vi "SocketHandle_1 - 複製.vi"(7 "Mode":enum16{"Open", "Read", "Write", "Close"}(ring), 8 "error in (no error)":errorcluster, 9 "data in":string, 10 "Port":u16=6342, 11 "Machine":string="localhost") -> (0 "error out":errorcluster, 3 "data out":string)   [LabVIEW 2011]
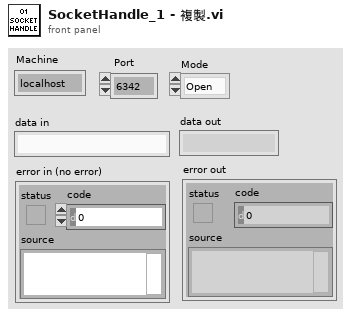
[diagram p1: front panel]
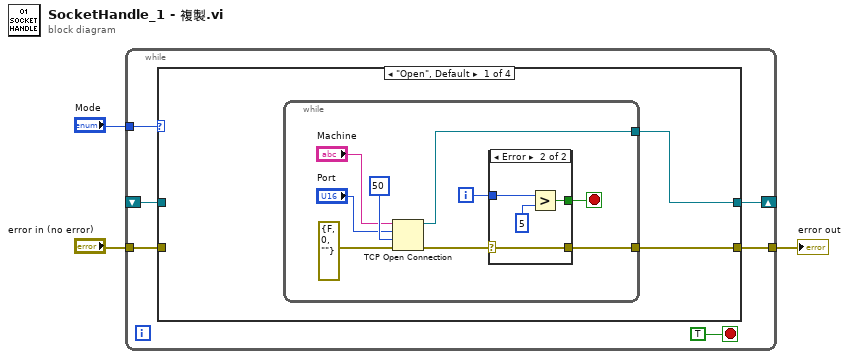
[diagram p0: block diagram]
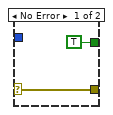
[diagram p2: hidden frame]
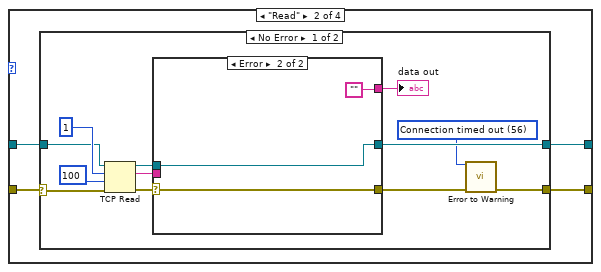
[diagram p3: hidden frame]
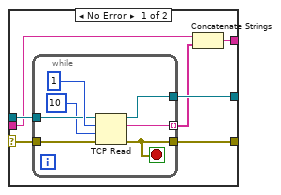
[diagram p4: hidden frame]
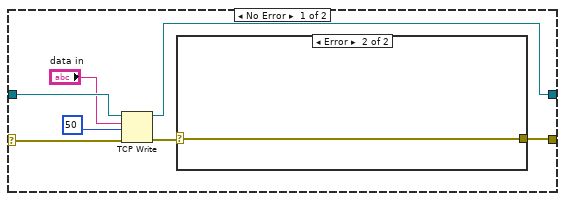
[diagram p7: hidden frame]
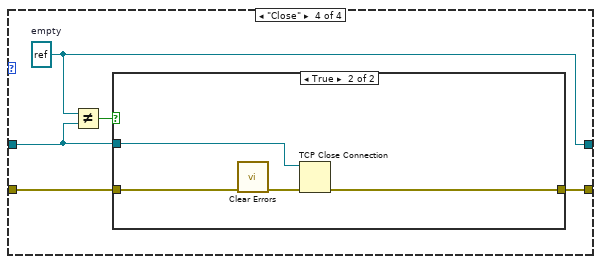
[diagram p9: hidden frame]
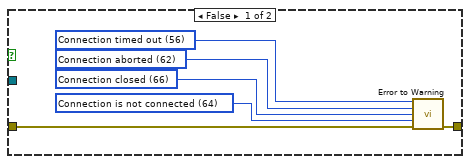
[diagram p10: hidden frame]
diagram:
  n1 = while {
    shift-right: [w9] -> _
    shift-left: _ -> [w6]
    tunnel: "Mode" -> [w5]
    tunnel: "error in (no error)" -> [w7]
    tunnel: [w8] -> w1
    stop <- TRUE stop-if-true
    n2 = case shown="\"Open\", Default" w5 {
      tunnel: [w11 w30 w64 w77] -> w9
      tunnel: [w10 w27 w63 w81] -> w8
      tunnel: w7 -> [_ w28 w62 w80]
      tunnel: w6 -> [_ w29 w65 w78]
      frame "Open", Default {
        n3 = while {
          tunnel: [w20] -> w11
          tunnel: [w15] -> w10
          i -> [w13]
          stop <- w12 stop-if-true
          n4 = TCP Open Connection(address="Machine", remote port or service name="Port", timeout ms (60000)=50, error in (no error)=errorcluster {"status"=FALSE, "code"=0, "source"=""} ("error constant")) -> (connection ID=w20:refnum<k5>, error out=w14:errorcluster)  [unwired: 1 out]
          n5 = case shown="Error" w14 {
            selector: w14 -> [w21 w26]
            tunnel: [w21 w26] -> w15
            tunnel: w13 -> [_ w25]
            tunnel: [TRUE w23] -> w12
            frame No Error {
            }
            frame Error {
              n6 = Greater?(x=w25, y=5) -> (0:w23:bool)
            }
          }
        }
      }
      frame "Read" {
        n7 = case shown="No Error" w28 {
          selector: w28 -> [w34 w60]
          tunnel: [w31 w60] -> w27
          tunnel: [w37 w61] -> w30
          tunnel: w29 -> [w36 w61]
          frame No Error {
            w33 = 56 items=["No Error", "Argument Error", "Memory Full", "Out of Zone", "End of File", "File Already Open", "Generic File IO Error", "File Not Found", "File Permission Error", "Disk Full", "Duplicate Path", "Too Many Files Open", "Not Enabled", "Resource File Not Found", "Cannot Add Resource", "Resource Not Found", "Image Not Found", "Image Memory Error", "Pen Does Not Exist", "Config Bad Type", "Config Token Not Found", "Config Parse Error", "Config Memory Error", "Bad External Code Format", "Bad External Code Offset", "External Code Not Present", "Null Window", "Destroy Window Mixup", "Null Menu", "Print Aborted", "Bad Print Record", "Print Driver Error", "Windows Error During Print", "Memory Error During Print", "Print Dialog Error", "Generic Print Error", "Invalid Device Refnum", "Device Not Found", "Device Parameter Error", "Device Unit Error", "Can't Open Device", "Device Call Aborted", "Generic Error", "Cancelled By User", "Object ID Too Low", "Object ID Too High", "Object Not In Heap", "Unknown Heap", "Bad DefProc ID", "DefProc Not In Table", "Message Out Of Range", "Null Method", "Unknown Message", "Manager Call Not Supported", "Bad address", "Connection In progress", "Connection timed out", "Connection is already in progress", "Network attribute not supported", "Network error", "Address in use", "System out of memory", "Connection aborted", "Connection refused", "Connection is not connected", "Connection is already connected", "Connection closed", "Initialize error (interapplication manager)", "Bad occurrence", "Wait on unbound occurrence handler", "Occurrence queue overflow", "Bad path", "Semaphore not signaled", "Unrecognized type (interapplication manager)"] ("1st Error to Convert")
            n8 = TCP Read(connection ID=w36, bytes to read=1, error in (no error)=w34, 9:100 ("timeout ms (25000)")) -> (connection ID out=w41:refnum<k5>, data out=w42:string, error out=w39:errorcluster)  [unwired: 1 in]
            n9 = case shown="Error" w39 {
              selector: w39 -> [w49 w58]
              tunnel: w42 -> [w44 _]
              tunnel: w41 -> [w48 w59]
              tunnel: [w47 w59] -> w37
              tunnel: [w46 ""] -> w35
              tunnel: [w43 w58] -> w32
              frame No Error {
                n10 = while {
                  tunnel: w49 -> [w56]
                  tunnel: w48 -> [w54]
                  tunnel: [w53] -> w47
                  tunnel: [w52] -> w45 mode=indexing
                  tunnel: [w51] -> w43
                  stop <- w51 stop-if-true
                  n11 = TCP Read(connection ID=w54, bytes to read=1, error in (no error)=w56, 9:10 ("timeout ms (25000)")) -> (connection ID out=w53:refnum<k5>, data out=w52:string, error out=w51:errorcluster)  [unwired: 1 in]
                }
                n12 = Concatenate Strings(w44, w45) -> (w46:string)
              }
              frame Error {
              }
            }
            "data out" <- w35
            n13 = call <vilib>:"Error to Warning.vi"("1st Error to Convert"=w33, "error in"=w32) -> ("warning out"=w31:errorcluster)  [unwired: 13 in]
          }
          frame Error {
          }
        }
      }
      frame "Write" {
        n14 = case shown="Error" w62 {
          selector: w62 -> [w70 w75]
          tunnel: w65 -> [w72 w76]
          tunnel: [w66 w76] -> w64
          tunnel: [w67 w75] -> w63
          frame No Error {
            n15 = TCP Write(connection ID=w72, data in="data in", error in (no error)=w70, 9:50 ("timeout ms (25000)")) -> (connection ID out=w66:refnum<k5>, error out=w68:errorcluster)  [unwired: 1 out]
            n16 = case shown="Error" w68 {
              selector: w68 -> [w73 w74]
              tunnel: [w73 w74] -> w67
              frame No Error {
              }
              frame Error {
              }
            }
          }
          frame Error {
          }
        }
      }
      frame "Close" {
        w77 = refnum<k5> refnum  # empty
        n17 = Not Equal?(x=w77, y=w78) -> (x != y?=w79:bool)
        n18 = case shown="True" w79 {
          tunnel: [w86 w91] -> w81
          tunnel: w80 -> [w87 w90]
          tunnel: w78 -> [_ w88]
          frame False {
            w82 = 64 items=["No Error", "Argument Error", "Memory Full", "Out of Zone", "End of File", "File Already Open", "Generic File IO Error", "File Not Found", "File Permission Error", "Disk Full", "Duplicate Path", "Too Many Files Open", "Not Enabled", "Resource File Not Found", "Cannot Add Resource", "Resource Not Found", "Image Not Found", "Image Memory Error", "Pen Does Not Exist", "Config Bad Type", "Config Token Not Found", "Config Parse Error", "Config Memory Error", "Bad External Code Format", "Bad External Code Offset", "External Code Not Present", "Null Window", "Destroy Window Mixup", "Null Menu", "Print Aborted", "Bad Print Record", "Print Driver Error", "Windows Error During Print", "Memory Error During Print", "Print Dialog Error", "Generic Print Error", "Invalid Device Refnum", "Device Not Found", "Device Parameter Error", "Device Unit Error", "Can't Open Device", "Device Call Aborted", "Generic Error", "Cancelled By User", "Object ID Too Low", "Object ID Too High", "Object Not In Heap", "Unknown Heap", "Bad DefProc ID", "DefProc Not In Table", "Message Out Of Range", "Null Method", "Unknown Message", "Manager Call Not Supported", "Bad address", "Connection In progress", "Connection timed out", "Connection is already in progress", "Network attribute not supported", "Network error", "Address in use", "System out of memory", "Connection aborted", "Connection refused", "Connection is not connected", "Connection is already connected", "Connection closed", "Initialize error (interapplication manager)", "Bad occurrence", "Wait on unbound occurrence handler", "Occurrence queue overflow", "Bad path", "Semaphore not signaled", "Unrecognized type (interapplication manager)"] ("1st Error to Convert")
            w83 = 66 items=["No Error", "Argument Error", "Memory Full", "Out of Zone", "End of File", "File Already Open", "Generic File IO Error", "File Not Found", "File Permission Error", "Disk Full", "Duplicate Path", "Too Many Files Open", "Not Enabled", "Resource File Not Found", "Cannot Add Resource", "Resource Not Found", "Image Not Found", "Image Memory Error", "Pen Does Not Exist", "Config Bad Type", "Config Token Not Found", "Config Parse Error", "Config Memory Error", "Bad External Code Format", "Bad External Code Offset", "External Code Not Present", "Null Window", "Destroy Window Mixup", "Null Menu", "Print Aborted", "Bad Print Record", "Print Driver Error", "Windows Error During Print", "Memory Error During Print", "Print Dialog Error", "Generic Print Error", "Invalid Device Refnum", "Device Not Found", "Device Parameter Error", "Device Unit Error", "Can't Open Device", "Device Call Aborted", "Generic Error", "Cancelled By User", "Object ID Too Low", "Object ID Too High", "Object Not In Heap", "Unknown Heap", "Bad DefProc ID", "DefProc Not In Table", "Message Out Of Range", "Null Method", "Unknown Message", "Manager Call Not Supported", "Bad address", "Connection In progress", "Connection timed out", "Connection is already in progress", "Network attribute not supported", "Network error", "Address in use", "System out of memory", "Connection aborted", "Connection refused", "Connection is not connected", "Connection is already connected", "Connection closed", "Initialize error (interapplication manager)", "Bad occurrence", "Wait on unbound occurrence handler", "Occurrence queue overflow", "Bad path", "Semaphore not signaled", "Unrecognized type (interapplication manager)"] ("1st Error to Convert")
            w84 = 62 items=["No Error", "Argument Error", "Memory Full", "Out of Zone", "End of File", "File Already Open", "Generic File IO Error", "File Not Found", "File Permission Error", "Disk Full", "Duplicate Path", "Too Many Files Open", "Not Enabled", "Resource File Not Found", "Cannot Add Resource", "Resource Not Found", "Image Not Found", "Image Memory Error", "Pen Does Not Exist", "Config Bad Type", "Config Token Not Found", "Config Parse Error", "Config Memory Error", "Bad External Code Format", "Bad External Code Offset", "External Code Not Present", "Null Window", "Destroy Window Mixup", "Null Menu", "Print Aborted", "Bad Print Record", "Print Driver Error", "Windows Error During Print", "Memory Error During Print", "Print Dialog Error", "Generic Print Error", "Invalid Device Refnum", "Device Not Found", "Device Parameter Error", "Device Unit Error", "Can't Open Device", "Device Call Aborted", "Generic Error", "Cancelled By User", "Object ID Too Low", "Object ID Too High", "Object Not In Heap", "Unknown Heap", "Bad DefProc ID", "DefProc Not In Table", "Message Out Of Range", "Null Method", "Unknown Message", "Manager Call Not Supported", "Bad address", "Connection In progress", "Connection timed out", "Connection is already in progress", "Network attribute not supported", "Network error", "Address in use", "System out of memory", "Connection aborted", "Connection refused", "Connection is not connected", "Connection is already connected", "Connection closed", "Initialize error (interapplication manager)", "Bad occurrence", "Wait on unbound occurrence handler", "Occurrence queue overflow", "Bad path", "Semaphore not signaled", "Unrecognized type (interapplication manager)"] ("1st Error to Convert")
            w85 = 56 items=["No Error", "Argument Error", "Memory Full", "Out of Zone", "End of File", "File Already Open", "Generic File IO Error", "File Not Found", "File Permission Error", "Disk Full", "Duplicate Path", "Too Many Files Open", "Not Enabled", "Resource File Not Found", "Cannot Add Resource", "Resource Not Found", "Image Not Found", "Image Memory Error", "Pen Does Not Exist", "Config Bad Type", "Config Token Not Found", "Config Parse Error", "Config Memory Error", "Bad External Code Format", "Bad External Code Offset", "External Code Not Present", "Null Window", "Destroy Window Mixup", "Null Menu", "Print Aborted", "Bad Print Record", "Print Driver Error", "Windows Error During Print", "Memory Error During Print", "Print Dialog Error", "Generic Print Error", "Invalid Device Refnum", "Device Not Found", "Device Parameter Error", "Device Unit Error", "Can't Open Device", "Device Call Aborted", "Generic Error", "Cancelled By User", "Object ID Too Low", "Object ID Too High", "Object Not In Heap", "Unknown Heap", "Bad DefProc ID", "DefProc Not In Table", "Message Out Of Range", "Null Method", "Unknown Message", "Manager Call Not Supported", "Bad address", "Connection In progress", "Connection timed out", "Connection is already in progress", "Network attribute not supported", "Network error", "Address in use", "System out of memory", "Connection aborted", "Connection refused", "Connection is not connected", "Connection is already connected", "Connection closed", "Initialize error (interapplication manager)", "Bad occurrence", "Wait on unbound occurrence handler", "Occurrence queue overflow", "Bad path", "Semaphore not signaled", "Unrecognized type (interapplication manager)"] ("1st Error to Convert")
            n19 = call <vilib>:"Error to Warning.vi"("1st Error to Convert"=w85, "2nd Error to Convert"=w84, "3rd Error to Convert"=w83, "4th Error to Convert"=w82, "error in"=w87) -> ("warning out"=w86:errorcluster)  [unwired: 10 in]
          }
          frame True {
            n20 = call <vilib>:"Clear Errors.vi"("error in (no error)"=w90) -> ("error out"=w89:errorcluster)  [unwired: 6 in]
            n21 = TCP Close Connection(connection ID=w88, error in (no error)=w89) -> (error out=w91:errorcluster)  [unwired: 2 out]
          }
        }
      }
    }
  }
  "error out" <- w1
